vi "Get Type.vi"(8 "error in (no error)":errorcluster, 11 "Wooden Case in":refnum<class "Wooden Case.lvclass">) -> (0 "error out":errorcluster, 2 "Item Type":T1, 3 "Wooden Case out":refnum<class "Wooden Case.lvclass">)   [LabVIEW 2020, in "Wooden Case.lvclass"]
uses:
  Wooden Case.lvclass
  Item/Item Type.ctl
  Item/Item.lvclass
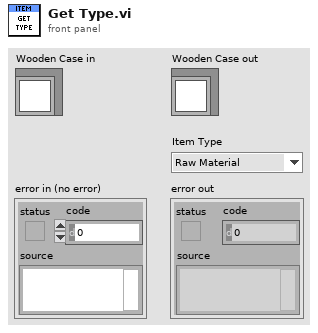
[diagram p1: front panel]
types:
  T1 = typedef "Item.lvclass/Item Type.ctl" = enum16{"Raw Material", "Component", "Module", "Product"}
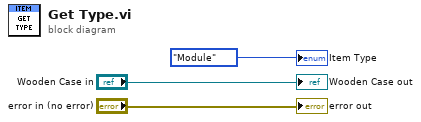
[diagram p0: block diagram]
diagram:
  "error out" <- "error in (no error)"
  "Wooden Case out" <- "Wooden Case in"
  "Item Type" <- Item_Type."Module" ("Item Type")
